vi "getEvaluation.vi"(8 "error in (no error)":errorcluster, 11 "TreeNode in":refnum<class "TreeNode.lvclass">) -> (0 "error out":errorcluster, 2 "evaluation":cluster{"F":dbl, "G":dbl, "H":dbl}, 3 "TreeNode out":refnum<class "TreeNode.lvclass">)   [LabVIEW 2010, in "TreeNode.lvclass"]
doc: "Gets the numerical evaluation of a node during a search."
uses:
  TreeNode.lvclass
  TreeNode.lvclass/TreeNode.ctl
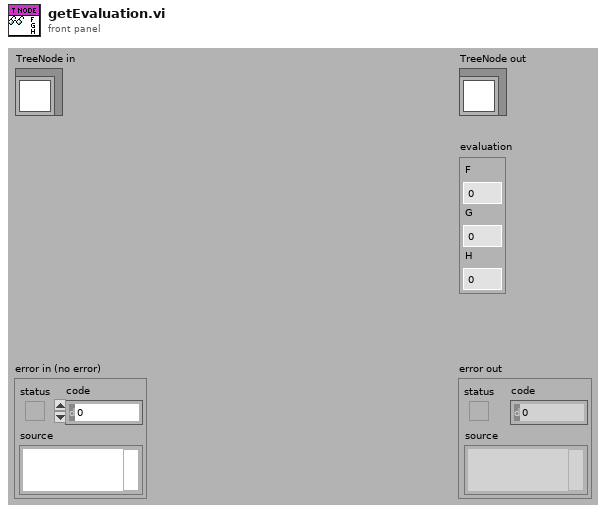
[diagram p1: front panel]
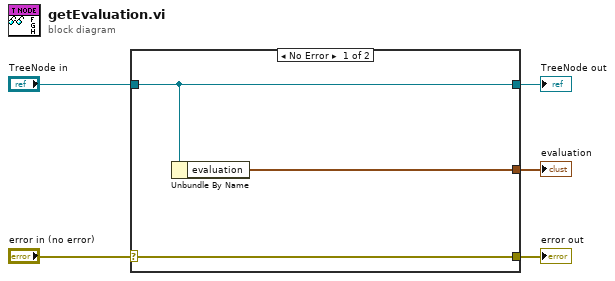
[diagram p0: block diagram]
diagram:
  n1 = case shown="No Error" "error in (no error)" {
    selector: "error in (no error)" -> [w8 w9]
    tunnel: [w8 w9] -> w4
    tunnel: [w7 w10] -> w2
    tunnel: "TreeNode in" -> [w7 w10]
    tunnel: [w6 _] -> w1
    frame No Error {
      n2 = Unbundle By Name(w7) -> ("evaluation"=w6:cluster{"F":dbl, "G":dbl, "H":dbl})
    }
    frame Error {
    }
  }
  "error out" <- w4
  "TreeNode out" <- w2
  "evaluation" <- w1
